vi "GenerateCode.vi"(1 "Terms":T1[](array[typedef]), 3 "Diagram":refnum<vi>, 5 "XRef":refnum<vi>, 6 "State In":T4) -> (0 "Generated Code?":bool, 2 "State Out":T4, 4 "Reply":string[](array[string]))   [LabVIEW 2012, in "Minimum Array Size.xnode"]
uses:
  Minimum Array Size.xnode
  State.ctl
  <vilib>/XNodeSupport/XNodeTermIDPair.ctl
  <vilib>/XNodeSupport/XNodeTermRef.ctl
  <vilib>/XNodeSupport/XNodeString.ctl
  <vilib>/Utility/miscctls.llb/LVPositionTypeDef.ctl
  <vilib>/Utility/miscctls.llb/LVPointTypeDef.ctl
  <userlib>/_LAVAcr/Scripting Tools/Scripting Tools.lvlib
  <vilib>/Utility/VariantDataType/VariantType.lvlib
  <vilib>/XNodeSupport/NI_XNodeSupport.lvlib
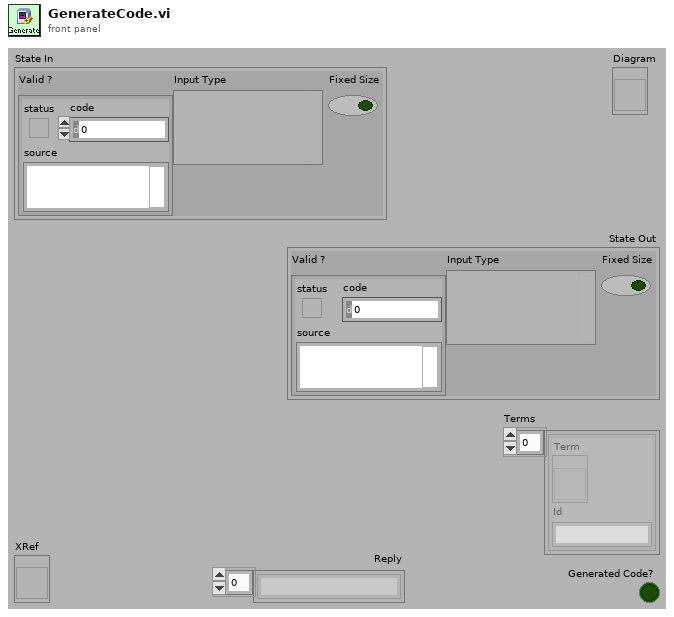
[diagram p1: front panel]
types:
  T1 = typedef "NI_XNodeSupport.lvlib/XNodeTermIDPair.ctl" = cluster{"Term":T2, "Id":T3}
  T2 = typedef "NI_XNodeSupport.lvlib/XNodeTermRef.ctl" = refnum<vi>
  T3 = typedef "NI_XNodeSupport.lvlib/XNodeString.ctl" = string
  T4 = typedef "Minimum Array Size.xnode/State.ctl" = cluster{"Valid ?":errorcluster, "Input Type":variant, "Fixed Size":bool}
  T5 = typedef "LVPointTypeDef.ctl" = cluster{"Horizontal":i16, "Vertical":i16}
  T6 = typedef "LVPositionTypeDef.ctl" = cluster{"Left":i32, "Top":i32}
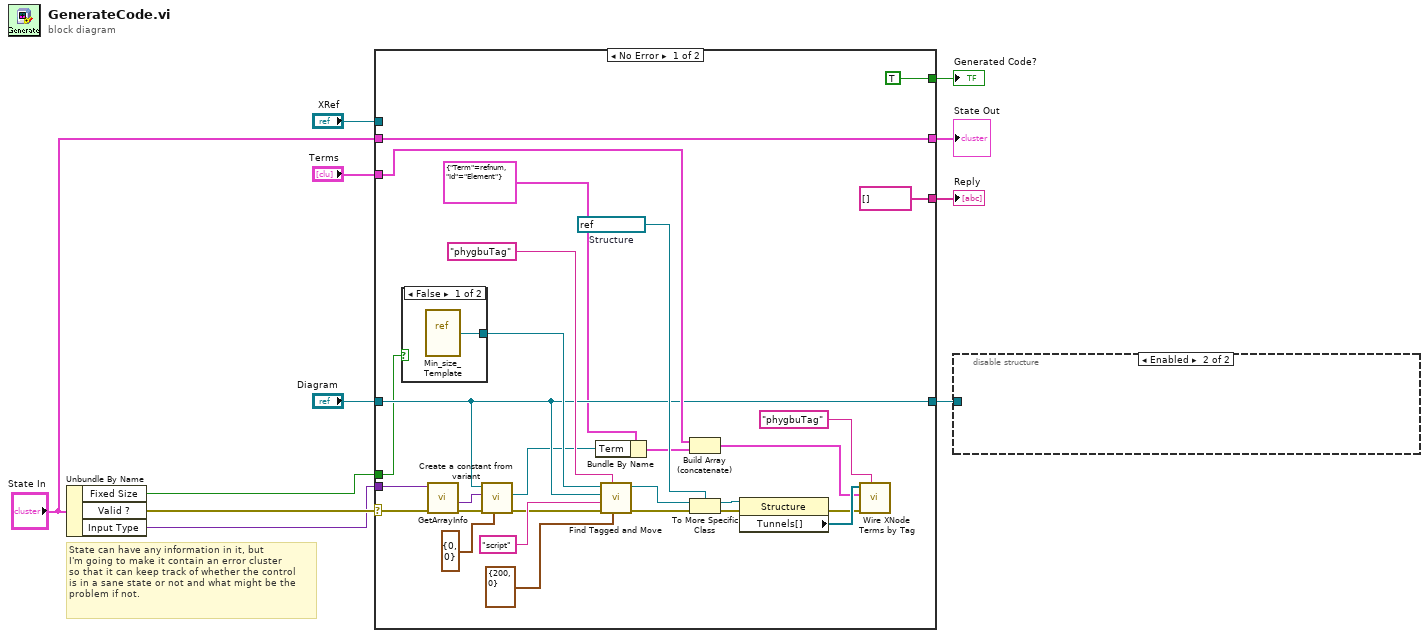
[diagram p0: block diagram]
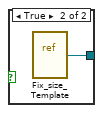
[diagram p2: hidden frame]
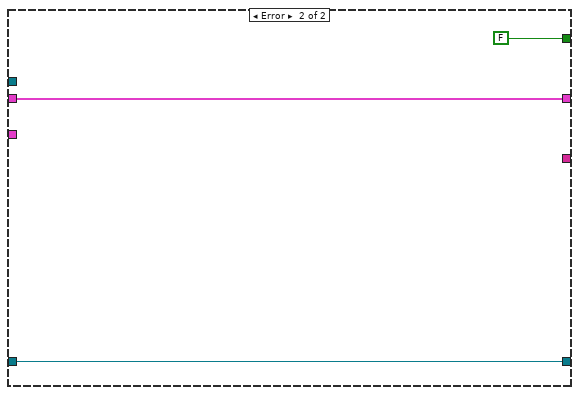
[diagram p3: hidden frame]
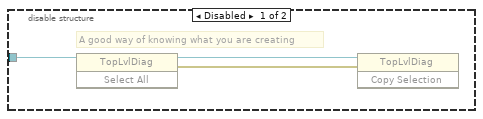
[diagram p4: hidden frame]
diagram:
  # "State can have any information in it, but\nI'm going to make it contain an error cluster\nso that it can keep track of whether the control\nis in a sane state or not and what might be the\nproblem if not."
  n1 = Unbundle By Name("State In") -> ("Fixed Size"=w1:bool, "Valid ?"=w11:errorcluster, "Input Type"=w2:variant)
  n2 = case shown="No Error" w11 {
    selector: w11 -> [w13 _]
    tunnel: "State In" -> [w37 w44]
    tunnel: "Diagram" -> [w22 w42]
    tunnel: "Terms" -> [w36 _]
    tunnel: "XRef" -> [_ _]
    tunnel: [w22 w42] -> w3
    tunnel: [string[] [] ("Reply") _] -> w6
    tunnel: [TRUE FALSE] -> w5
    tunnel: [w37 w44] -> w4
    tunnel: w2 -> [w23 _]
    tunnel: w1 -> [w14 _]
    frame No Error {
      w34 = refnum<vi> refnum  # Structure
      n3 = case shown="False" w14 {
        tunnel: [w40 w41] -> w24
        frame False {
          n4 = vi-ref "Min_size_Template.vi"() -> (w40:refnum<vi>)
        }
        frame True {
          n5 = vi-ref "Fix_size_Template.vi"() -> (w41:refnum<vi>)
        }
      }
      n6 = call <vilib>:"GetArrayInfo.vi"("error in (no error)"=w13, "Variant"=w23) -> ("error out"=w12:errorcluster, "ArrayElement"=w21:variant)  [unwired: 8 out]
      n7 = call <userlib>:"Create a constant from variant.vi"("relative position/next to refnum"=T5 {"Horizontal"=0, "Vertical"=0}, "error in (no error)"=w12, "Constant Data"=w21, "Diagram"=w22) -> ("error out"=w16:errorcluster, "Terminal"=w18:refnum<vi>)  [unwired: 1 in, 5 out]
      n8 = Bundle By Name(cluster=T1 {"Term"=refnum, "Id"="Element"} ("Code Gen Term"), "Term"=w18) -> (w17:T1)
      n9 = call <userlib>:"Find Tagged and Move.vi"("position"=T6 {"Left"=200, "Top"=0}, "TagName"="phygbuTag", "error in"=w16, "TagValue"="script", "Destination Diagram"=w22, "VI Refnum"=w24) -> ("error out"=w28:errorcluster, "Moved Tagged object"=w29:refnum<vi>)  [unwired: 4 out]
      n10 = Build Array (concatenate)(w36, w17) -> (w20:T1[])
      n11 = To More Specific Class(target class=w34, reference=w29, error in=w28) -> (specific class reference=w35:refnum<vi>, error out=w27:errorcluster)
      n12 = property class="Structure"(reference=w35, error in=w27) -> (error out=w26:errorcluster, "Tunnels[]"=w33:refnum<vi>[])  [unwired: 1 out]
      n13 = call <userlib>:"Wire XNode Terms by Tag.vi"("TagName"="phygbuTag", "error in (no error)"=w26, "Term Refs"=w20, "Source References"=w33) -> ()  [unwired: 8 out]
    }
    frame Error {
    }
  }
  "State Out" <- w4
  "Reply" <- w6
  "Generated Code?" <- w5
  n14 = disable-structure shown="Enabled" {
    disable-tunnel: w3 -> [w45 _]
    frame Disabled {
      # "A good way of knowing what you are creating"
      n15 = invoke class="TopLvlDiag" method="Select All"(reference=w45) -> (reference out=w47:refnum<vi>, error out=w46:errorcluster)  [unwired: 2 in, 1 out]
      n16 = invoke class="TopLvlDiag" method="Copy Selection"(reference=w47, error in=w46) -> ()  [unwired: 1 in, 3 out]
    }
    frame Enabled {
    }
  }
